vi "Is_TopLevel.vi"(8 "error in (no error)":errorcluster, 11 "AB_Source_ExportedVI in":refnum<class "AB_Source_ExportedVI.lvclass">) -> (0 "error out":errorcluster, 1 "openVIreference":bool, 2 "path":path, 3 "AB_Source_ExportedVI out":refnum<class "AB_Source_ExportedVI.lvclass">, 5 "readLinker":bool)   [LabVIEW 2020, in "AB_Source_ExportedVI.lvclass"]
uses:
  <vilib>/AppBuilder/AB_Classes/Source/ExportedVI/AB_Source_ExportedVI.lvclass
  e:/builds/penguin/labview/branches/2020/dev/dist/vi.lib/AppBuilder/AB_Classes/Source/AB_Source.lvclass
  e:/builds/penguin/labview/branches/2020/dev/dist/vi.lib/AppBuilder/AB_Classes/Source/VI/AB_Source_VI.lvclass
  <resource>/Framework/Providers/Common/provcom_StringGlobals.vi
  <vilib>/AppBuilder/AB_Classes/Source/VI/AB_Source_VI.lvclass
  <vilib>/AppBuilder/AB_Classes/Source/AB_Source.lvclass
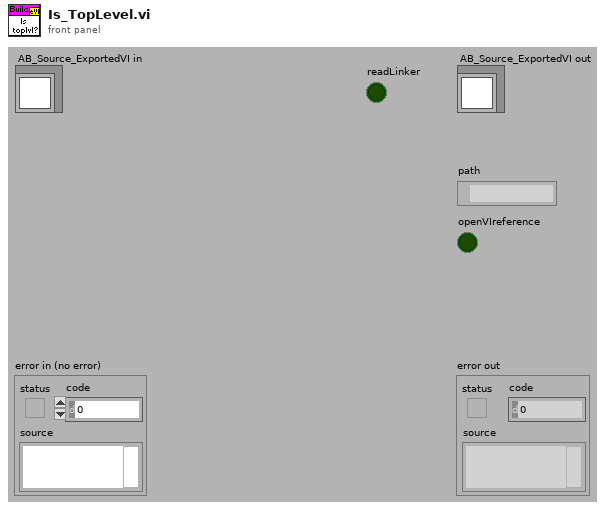
[diagram p1: front panel]
types:
  T1 = typedef "AB_Source.ctl" = cluster{"path":path, "itemID":string, "parentIndex":i32, "sourceInclusion":T2, "destinationIndex":i32, "properties":T3[], "newName":string, "lvfile":bool, "valid":bool, "eng_inBuild":bool, "eng_isNonVILink":bool, "Amalgamation":bool, "Amalgamation Piece":bool, "eng_delimitedName":string, "preventRename":bool}
  T2 = typedef "AB_Source_Inclusion.ctl" = enum16{"IncludeIfReferenced", "Include", "Exclude", "TopLevel"}
  T3 = typedef "AB_Source_Properties.ctl" = cluster{"sourcePropertyType":T4, "value":variant}
  T4 = typedef "AB_Source_Property_Type.ctl" = enum16{"Remove block diagram", "Remove front panel", "Password", "Window has title bar", "Show menu bar", "Show vertical scroll bar", "Show horizontal scroll bar", "Show toolbar", "Show Abort button", "Show fp when called", "Window behavior", "Allow user to close window", "Window run-time position", "Run when opened", "Allow debugging", "Auto error handling", "Generate guard code", "Use stack variables", "Expression folding", "Integer only", "Inline subVI"}
  T5 = typedef "AB_Source_VI.ctl" = cluster{"standardVI":bool, "dynamicDispatch":bool, "LLBtopLevel":bool, "privateDataControl":bool, "eng_hasNonVILinks":bool, "eng_reference":refnum<vi>, "eng_saveLevel":u32}
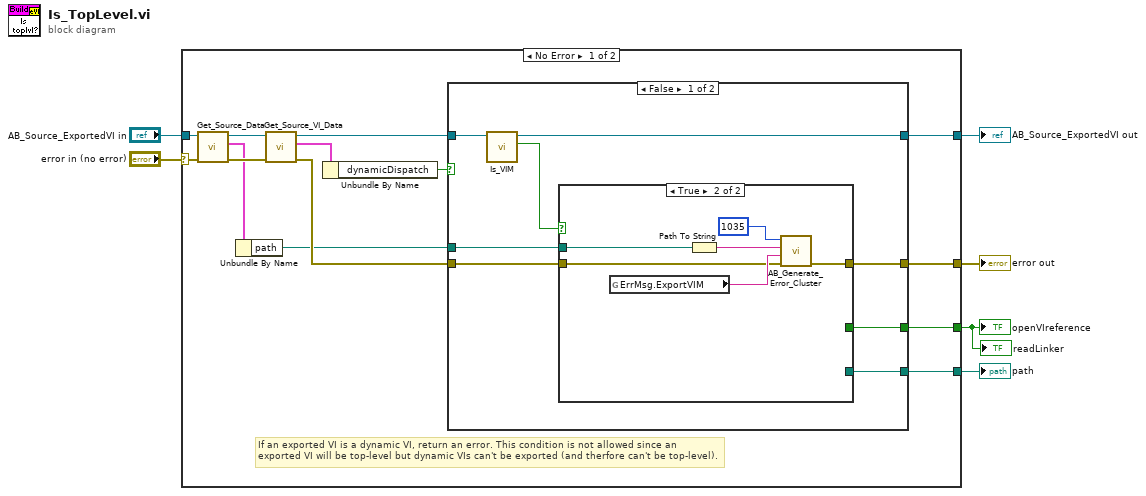
[diagram p0: block diagram]
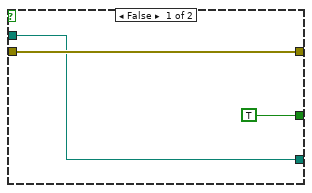
[diagram p2: hidden frame]
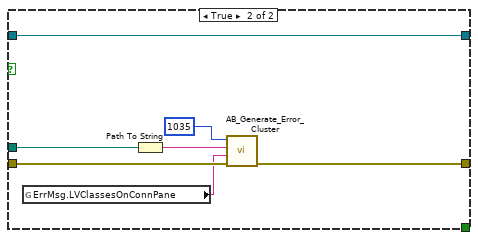
[diagram p3: hidden frame]
diagram:
  n1 = case shown="No Error" "error in (no error)" {
    selector: "error in (no error)" -> [w9 w45]
    tunnel: [w7 w46] -> w6
    tunnel: [w17 w45] -> w5
    tunnel: "AB_Source_ExportedVI in" -> [w14 w46]
    tunnel: [w11 _] -> w3
    tunnel: [w10 _] -> w2
    frame No Error {
      # "If an exported VI is a dynamic VI, return an error. This condition is not allowed since an exported VI will be top-level but dynamic VIs can't be exported (and therfore can't be top-level)."
      n2 = call <vilib>:"Get_Source_Data.vi"("error in (no error)"=w9, "Class in"=w14) -> ("error out"=w15:errorcluster, "data"=w13:T1, "Class out"=w16:refnum<class "AB_Source_ExportedVI.lvclass">)  [unwired: 7 out]
      n3 = Unbundle By Name(w13) -> ("path"=w12:path)
      n4 = call <vilib>:"Get_Source_VI_Data.vi"("error in (no error)"=w15, "Class in"=w16) -> ("error out"=w18:errorcluster, "data"=w20:T5, "Class out"=w8:refnum<class "AB_Source_ExportedVI.lvclass">)  [unwired: 7 out]
      n5 = Unbundle By Name(w20) -> ("dynamicDispatch"=w19:bool)
      n6 = case shown="False" w19 {
        tunnel: w18 -> [w25 w41]
        tunnel: [w24 w40] -> w17
        tunnel: w12 -> [w21 w42]
        tunnel: [w22 _] -> w11
        tunnel: [w23 _] -> w10
        tunnel: w8 -> [w28 w38]
        tunnel: [w27 w38] -> w7
        frame False {
          n7 = call-dynamic "Is_VIM.vi"("AB_Source_VI in"=w28) -> ("isVIM?"=w26:bool, "AB_Source_VI out"=w27:refnum<class "AB_Source_ExportedVI.lvclass">)  [unwired: 8 in, 1 out]
          n8 = case shown="True" w26 {
            tunnel: w25 -> [w30 w34]
            tunnel: [w30 w33] -> w24
            tunnel: [TRUE _] -> w23
            tunnel: [w29 _] -> w22
            tunnel: w21 -> [w29 w32]
            frame False {
            }
            frame True {
              n9 = global read "provcom_StringGlobals.vi" "ErrMsg.ExportVIM"() -> (w35:string)
              n10 = Path To String(path=w32) -> (string=w36:string)
              n11 = call <vilib>:"AB_Generate_Error_Cluster.vi"("error in (no error)"=w34, "Additional Message"=w35, "source"=w36, "Code"=1035 ("code")) -> ("error out"=w33:errorcluster)  [unwired: 7 out]
            }
          }
        }
        frame True {
          n12 = global read "provcom_StringGlobals.vi" "ErrMsg.LVClassesOnConnPane"() -> (w39:string)
          n13 = Path To String(path=w42) -> (string=w43:string)
          n14 = call <vilib>:"AB_Generate_Error_Cluster.vi"("error in (no error)"=w41, "Additional Message"=w39, "source"=w43, "Code"=1035 ("code")) -> ("error out"=w40:errorcluster)  [unwired: 7 out]
        }
      }
    }
    frame Error {
    }
  }
  "error out" <- w5
  "openVIreference" <- w2
  "path" <- w3
  "AB_Source_ExportedVI out" <- w6
  "readLinker" <- w2
